vi "UDP Data Link - Pages - Tx Channels Section Page.vi"(8 "error in (no error)":errorcluster, 11 "Node Ptr":T1 format="%.0x") -> (0 "error out":errorcluster)   [LabVIEW 2012, in "UDP Data Link System Explorer.lvlib"]
uses:
  UDP Data Link System Explorer.lvlib
  <vilib>/NI Veristand/Custom Device API/Custom Device Item Ref.ctl
  TypeDefs/UDP Data Link - TypeDefs - Tx Channels Section Page References.ctl
  Shared/UDP Data Link Global.vi
  <vilib>/NI Veristand/Custom Device API/Set Item Property (I32 Array).vi
  <vilib>/NI Veristand/Custom Device API/Custom Device API.lvlib
  Shared/UDP Data Link Shared.lvlib
panel:
  in  "Tx Channels":i32[](listbox)
  in  "Header":cluster{"Section Name":string}={"Section Name"="Transmit Settings"}
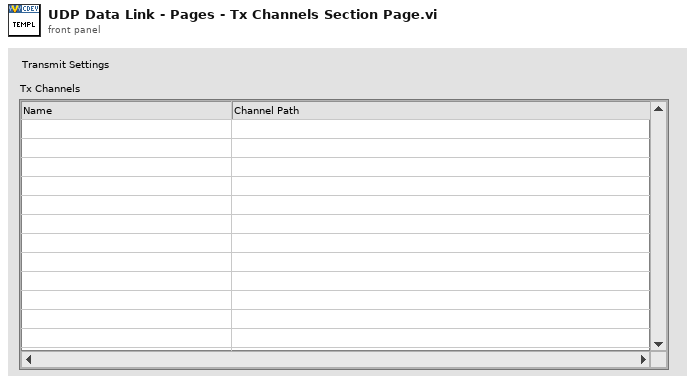
[diagram p1: front panel]
types:
  T1 = typedef "Custom Device API.lvlib/Custom Device Item Ref.ctl" = u64
  T2 = typedef "UDP Data Link System Explorer.lvlib/UDP Data Link - TypeDefs - Tx Channels Section Page References.ctl" = cluster{"Tx Channels":refnum<vi>}
  T3 = typedef "Custom Device API.lvlib/Custom Device Commands.ctl" = enum16{"Default", "Item renamed", "Shutdown", "Dynamic button pressed"}
  T4 = typedef "Custom Device API.lvlib/Custom Device Item Info.ctl" = cluster{"Name":string, "Is Channel":bool, "GUID":string, "Is Waveform":bool}
  T5 = typedef "LVPoint32TypeDef.ctl" = cluster{"Horizontal":i32, "Vertical":i32}
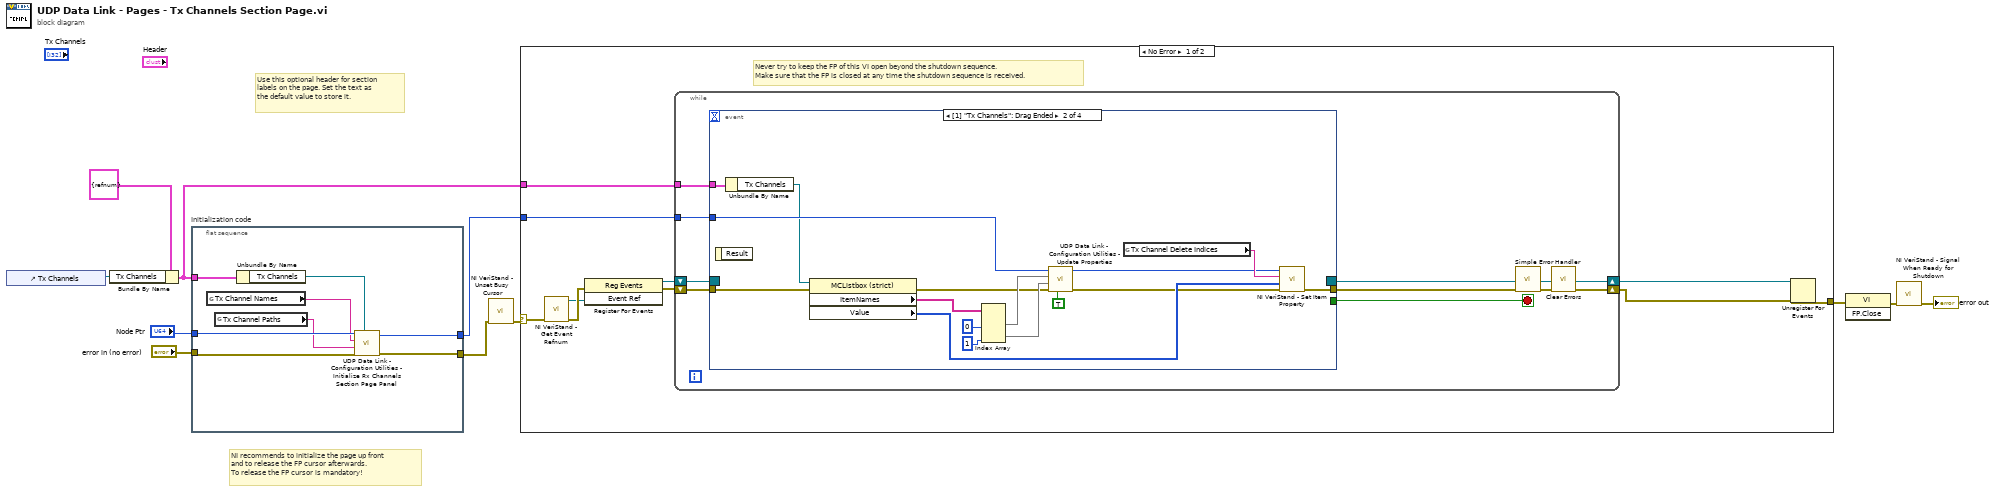
[diagram p0: block diagram]
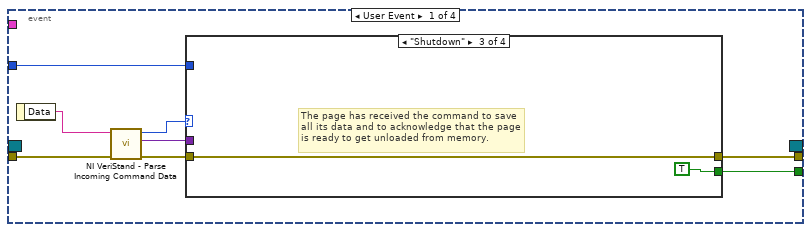
[diagram p2: hidden frame]
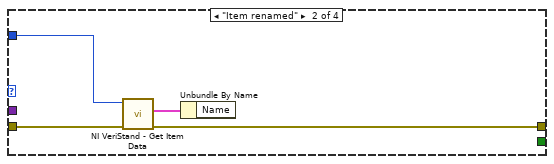
[diagram p4: hidden frame]
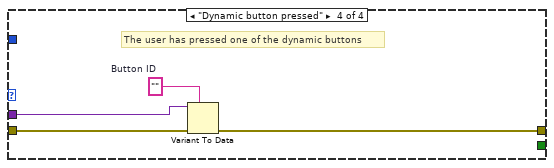
[diagram p5: hidden frame]
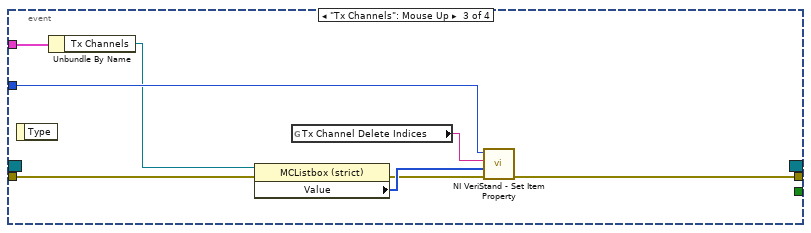
[diagram p6: hidden frame]
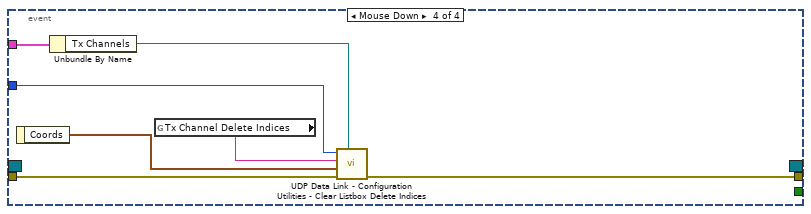
[diagram p7: hidden frame]
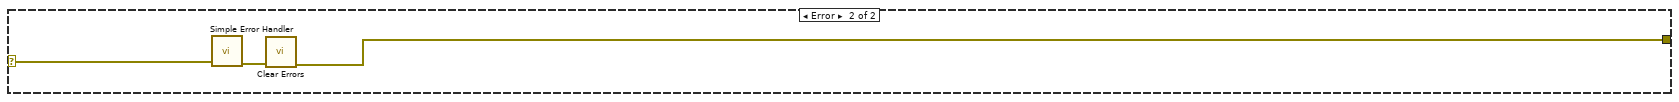
[diagram p8: hidden frame]
diagram:
  # "Use this optional header for section labels on the page. Set the text as the default value to store it."
  # "NI recommends to initialize the page up front\nand to release the FP cursor afterwards.\nTo release the FP cursor is mandatory!"
  n1 = control-ref of="Tx Channels"() -> (w3:refnum<vi>)
  n2 = Bundle By Name(cluster=T2 {"Tx Channels"=refnum} ("Tx Channels Section Cluster"), "Tx Channels"=w3) -> (w1:T2)
  n3 = flat-sequence "Initialization code" {
    tunnel: "error in (no error)" -> [w18]
    tunnel: "Node Ptr" -> [w16]
    tunnel: [w19] -> w7
    tunnel: [w17] -> w4
    tunnel: w1 -> [w13]
    frame #0 {
      n4 = global read "UDP Data Link Global.vi" "Tx Channel Names"() -> (w14:string)
      n5 = global read "UDP Data Link Global.vi" "Tx Channel Paths"() -> (w15:string)
      n6 = Unbundle By Name(w13) -> ("Tx Channels"=w12:refnum<vi>)
      n7 = call "UDP Data Link - Configuration Utilities - Initialize Rx Channels Section Page Panel.vi"("Channels Listbox"=w12, "error in (no error)"=w18, "Channel Paths Property"=w15, "Channel Names Property"=w14, "Item Ref in"=w16) -> ("error out"=w19:errorcluster, "Item Ref out"=w17:T1)  [unwired: 3 in, 2 out]
    }
  }
  n8 = call <vilib>:"NI VeriStand - Unset Busy Cursor.vi"("error in (no error)"=w7) -> ("error out"=w6:errorcluster)  [unwired: 10 out]
  n9 = case shown="No Error" w6 {
    selector: w6 -> [w21 w91]
    tunnel: [w26 w89] -> w11
    tunnel: w4 -> [w22 _]
    tunnel: w1 -> [w20 _]
    frame No Error {
      # "Never try to keep the FP of this VI open beyond the shutdown sequence.\nMake sure that the FP is closed at any time the shutdown sequence is received."
      n10 = call <vilib>:"NI VeriStand - Get Event Refnum.vi"("error in (no error)"=w21) -> ("error out"=w29:errorcluster, "Event Ref"=w25:refnum<user-event>)  [unwired: 9 out]
      n11 = register-events(error in=w29, w25) -> (reference out=w23:refnum<event-registration>, error out=w24:errorcluster)  [unwired: 1 in]
      n12 = while {
        tunnel: w22 -> [w34]
        shift-right: [w32] -> w27
        shift-left: w24 -> [w37]
        shift-right: [w38] -> w28
        shift-left: w23 -> [w36]
        tunnel: w20 -> [w30]
        stop <- w35 stop-if-true
        n13 = event shown="[1] \"Tx Channels\": Drag Ended" {
          selector: w36 -> [_ _ _ _]
          dyn-events: [_ _ _ _] -> w38
          timeout: _ -> [_ _ _ _]
          tunnel: w37 -> [w46 w61 w76 w86]
          tunnel: [w42 _ _ _] -> w35
          tunnel: [w41 w67 w80 w85] -> w31
          tunnel: w34 -> [w40 w73 w79 w83]
          tunnel: w30 -> [_ w65 w78 w87]
          event User Event {
            n14 = event-data() -> ("Data"=w45:string)  [unwired: 1 out]
            n15 = call <vilib>:"NI VeriStand - Parse Incoming Command Data.vi"("error in (no error)"=w46, "Incoming data"=w45) -> ("error out"=w44:errorcluster, "Outgoing data"=w39:variant, "Action"=w43:T3)  [unwired: 7 out]
            n16 = case shown="\"Shutdown\"" w43 {
              tunnel: w44 -> [w47 w51 w52 w57]
              tunnel: [_ _ TRUE _] -> w42
              tunnel: [w47 w48 w52 w54] -> w41
              tunnel: w40 -> [_ w50 _ _]
              tunnel: w39 -> [_ _ _ w56]
              frame "Default", Default {
              }
              frame "Item renamed" {
                n17 = call <vilib>:"NI VeriStand - Get Item Data.vi"("error in (no error)"=w51, "Item Ref in"=w50) -> ("error out"=w48:errorcluster, "Item Info"=w49:T4)  [unwired: 8 out]
                n18 = Unbundle By Name(w49) -> ()  [unwired: 1 out]
              }
              frame "Shutdown" {
                # "The page has received the command to save all its data and to acknowledge that the page is ready to get unloaded from memory."
              }
              frame "Dynamic button pressed" {
                w55 = ""  # Button ID
                # "The user has pressed one of the dynamic buttons"
                n19 = Variant To Data(error in=w57, type=w55, Variant=w56) -> (error out=w54:errorcluster)  [unwired: 1 out]
              }
            }
          }
          event "Tx Channels": Drag Ended {
            n20 = event-data() -> ()  [unwired: 2 out]
            n21 = Unbundle By Name(w65) -> ("Tx Channels"=w59:refnum<vi>)
            n22 = property class="MCListbox (strict)"(reference=w59, error in=w61) -> (error out=w60:errorcluster, "ItemNames"=w64:string[][], "Value"=w63:i32[])  [unwired: 1 out]
            n23 = Index Array(array=w64, index (col) #1=0 ("disabled index (col)"), index (col) #2=1 ("index (col)")) -> (element #1=w70:string[], element #2=w69:string[])  [unwired: 2 in]
            n24 = call "UDP Data Link - Configuration Utilities - Update Properties.vi"("Tx?"=TRUE, "error in (no error)"=w60, "Channel Paths"=w69, "Channel Names"=w70, "Item Ref in"=w73) -> ("error out"=w62:errorcluster, "Item Ref out"=w66:T1)  [unwired: 5 in]
            n25 = global read "UDP Data Link Global.vi" "Tx Channel Delete Indices"() -> (w68:string)
            n26 = call-poly <vilib>:"NI VeriStand - Set Item Property.vi"("error in (no error)"=w62, "Value"=w63, "Property Name"=w68, "Item Ref in"=w66) -> ("error out"=w67:errorcluster)  [unwired: 5 in, 2 out]
          }
          event "Tx Channels": Mouse Up {
            n27 = event-data() -> ()  [unwired: 2 out]
            n28 = Unbundle By Name(w78) -> ("Tx Channels"=w74:refnum<vi>)
            n29 = property class="MCListbox (strict)"(reference=w74, error in=w76) -> (error out=w75:errorcluster, "Value"=w77:i32[])  [unwired: 1 out]
            n30 = global read "UDP Data Link Global.vi" "Tx Channel Delete Indices"() -> (w81:string)
            n31 = call-poly <vilib>:"NI VeriStand - Set Item Property.vi"("error in (no error)"=w75, "Value"=w77, "Property Name"=w81, "Item Ref in"=w79) -> ("error out"=w80:errorcluster)  [unwired: 5 in, 2 out]
          }
          event Mouse Down {
            n32 = event-data() -> ("Coords"=w82:T5)  [unwired: 1 out]
            n33 = Unbundle By Name(w87) -> ("Tx Channels"=w84:refnum<vi>)
            n34 = global read "UDP Data Link Global.vi" "Tx Channel Delete Indices"() -> (w88:string)
            n35 = call "UDP Data Link - Configuration Utilities - Clear Listbox Delete Indices.vi"("Listbox Reference in"=w84, "error in (no error)"=w86, "Pane Coords"=w82, "Delete Property Name"=w88, "Item Ref in"=w83) -> ("error out"=w85:errorcluster)  [unwired: 5 in, 1 out]
          }
        }
        n36 = call <vilib>:"Simple Error Handler.vi"("error in (no error)"=w31) -> ("error out"=w33:errorcluster)  [unwired: 1 in, 7 out]
        n37 = call <vilib>:"Clear Errors.vi"("error in (no error)"=w33) -> ("error out"=w32:errorcluster)  [unwired: 6 out]
      }
      n38 = Unregister For Events(event registration refnum=w28, error in=w27) -> (error out=w26:errorcluster)
    }
    frame Error {
      n39 = call <vilib>:"Simple Error Handler.vi"("error in (no error)"=w91) -> ("error out"=w90:errorcluster)  [unwired: 1 in, 7 out]
      n40 = call <vilib>:"Clear Errors.vi"("error in (no error)"=w90) -> ("error out"=w89:errorcluster)  [unwired: 6 out]
    }
  }
  n41 = invoke class="VI" method="FP.Close"(error in=w11) -> (error out=w10:errorcluster)  [unwired: 2 in, 2 out]
  n42 = call <vilib>:"NI VeriStand - Signal When Ready for Shutdown.vi"("error in (no error)"=w10) -> ("error out"=→"error out":errorcluster)  [unwired: 10 out]
